vi "ScanCtrl_HR.vi"() -> ()   [LabVIEW 2020]
uses:
  C:/Users/MarcuLab/Desktop/V6 APD LV/V6 APD LV/Kinesis/Thorlabs.MotionControl.Controls.dll
  Kinesis/Thorlabs.MotionControl.Controls.dll
  <vilib>/event_ctls.llb/usereventprio.ctl
  C:/Users/MarcuLab/Desktop/V6 APD LV/V6 APD LV/Kinesis/Thorlabs.MotionControl.KCube.BrushlessMotorCLI.dll
  Kinesis/Thorlabs.MotionControl.KCube.BrushlessMotorCLI.dll
  C:/Users/MarcuLab/Desktop/V6 APD LV/V6 APD LV/Kinesis/ThorLabs.MotionControl.KCube.DCServoCLI.dll
  Kinesis/ThorLabs.MotionControl.KCube.DCServoCLI.dll
  C:/Users/MarcuLab/Desktop/V6 APD LV/V6 APD LV/Kinesis/Thorlabs.MotionControl.GenericMotorCLI.dll
  Kinesis/Thorlabs.MotionControl.GenericMotorCLI.dll
panel:
  out "error out":errorcluster
  out "TriggerPara":T1
  out "Trigger1Polarity":i32(ring)=1 items=["TriggerHigh"=1, "TriggerLow"=2]
  out "Trigger1Mode":i32(ring) items=["Disabled"=0, "TrigIN_GPI"=1, "TrigIN_RelativeMove"=2, "TrigIN_AbsoluteMove"=3, "TrigIN_Homed"=4, "TrigIN_Stop"=5, "TrigOUT_GPO"=10, "TrigOUT_InMotion"=11, "TrigOUT_AtMaxVelocity"=12, "TrigOUT_AtPositionFwd"=13, "TrigOUT_AtPositionRev"=14, "TrigOUT_AtPositionBoth"=15, "TrigOut_AtFwdLimit"=16, "TrigOut_AtBwdLimit"=17, "TrigOut_AtLimit"=18]
  in  "acceleration (mm/s2)":dbl=4000.0
  out "ScanRoute":cluster{dbl[], dbl[]}(graph)
  out "# of lines":u32
  in  "Start Scan":bool
  in  "Comp Scan Para":bool
  out "X speed (mm/s)":dbl format="%.4g"
  in  "Laser Rate (Hz)":u16=2500
  in  "Y step size (um)":dbl=10.0
  in  "X step size (um)":dbl=10.0
  in  "Y scan distance (mm)":dbl=0.2
  in  "X scan distance (mm)":dbl=30.0
  out "Y0 Position(mm)":dbl format="%.4g"
  out "GetPositionCounter 2":i32
  out "X0 Position(mm)":dbl format="%.4g"
  out "GetPositionCounter":i32
  in  "SetScanStart":bool
  in  "SerialNumber(Slow)":string="27000986"
  in  "SerialNumber(Fast)":string="28252795"
  in  "SlowAxis":refnum<k24>(container)
  in  "FastAxis":refnum<k24>(container)
  in  "Quit":bool
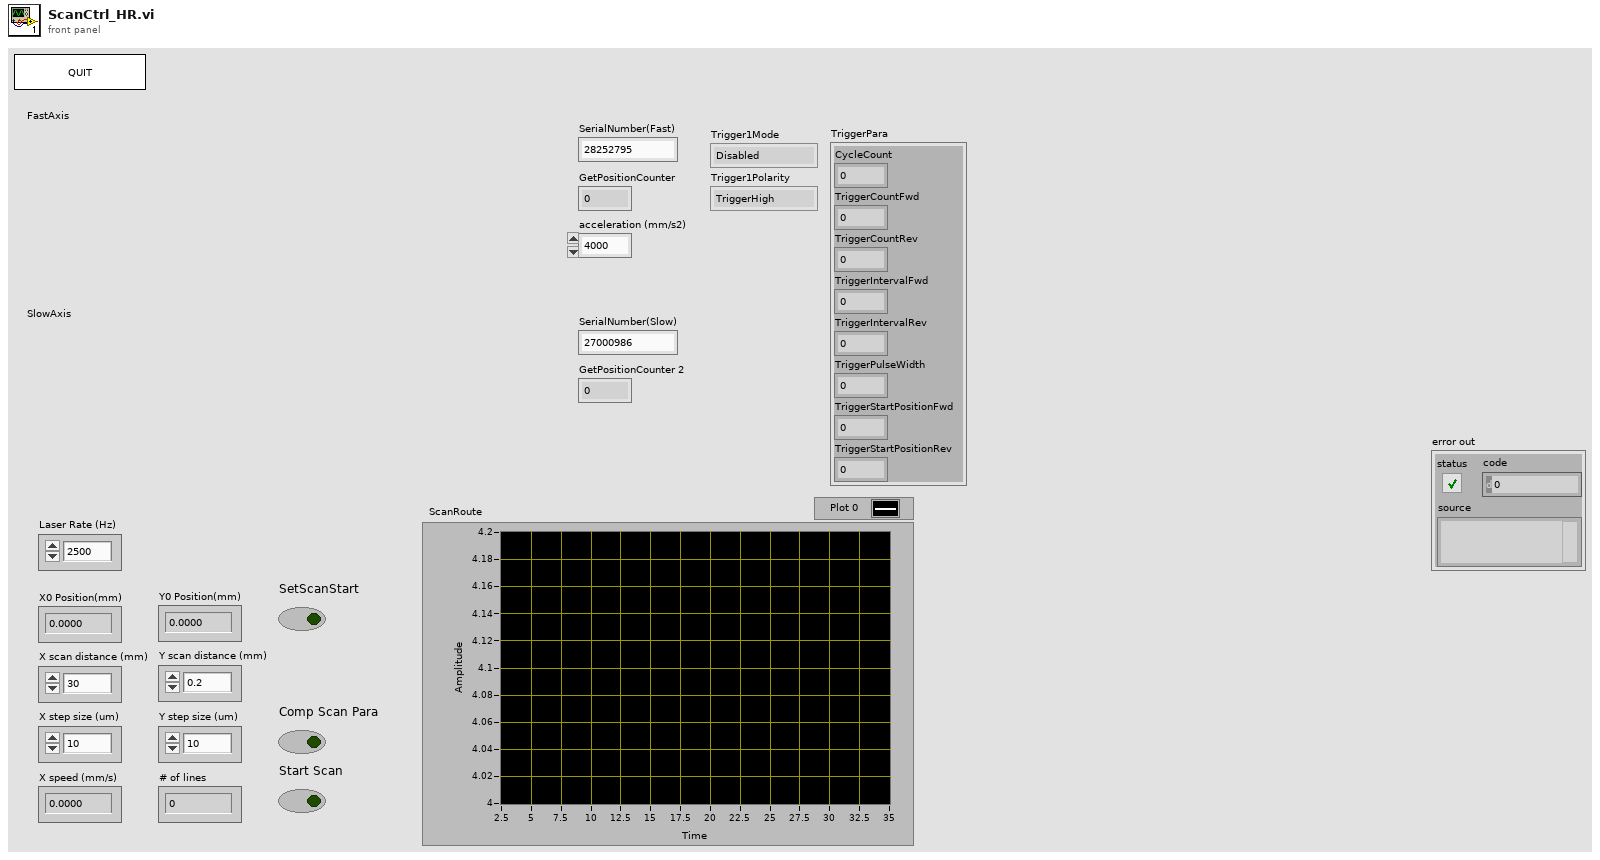
[diagram p1: front panel]
types:
  T1 = cluster{"CycleCount":i32, "TriggerCountFwd":i32, "TriggerCountRev":i32, "TriggerIntervalFwd":dbl, "TriggerIntervalRev":dbl, "TriggerPulseWidth":i32, "TriggerStartPositionFwd":dbl, "TriggerStartPositionRev":dbl}
  T2 = cluster{"X":dbl[], "Y":dbl[], "Device(Fast)":refnum<k24>, "Device(Slow)":refnum<k24>}
  T3 = enum32{"Invalid", "Standard", "Closed", "Hidden", "Minimized", "Maximized"}
  T4 = enum32{"invalid app kind", "Development System", "Run Time System", "Student Edition", "Embedded LabVIEW", "Evaluation", "Custom"}
  T5 = typedef "usereventprio.ctl" = enum32{"high priority", "normal priority"}
  T6 = enum16{"open", "open or create", "create or replace", "create", "open (read-only)"}
  T7 = cluster{"Core":cluster{"Current VI Reference":refnum<vi>, "Close Panel on Exit?":bool}, "FastAxisSerial":string, "SlowAxisSerial":string, "NetHandle(Fast)":refnum<k24>, "Device(Fast)":refnum<k24>, "NetHandle(Slow)":refnum<k24>, "Device(Slow)":refnum<k24>, "ScanRoute":cluster{dbl[], dbl[]}}
  T8 = cluster{"Current VI Reference":refnum<vi>, "Close Panel on Exit?":bool}
  T9 = cluster{"remote start event":refnum<user-event>, "remote stop event":refnum<user-event>}
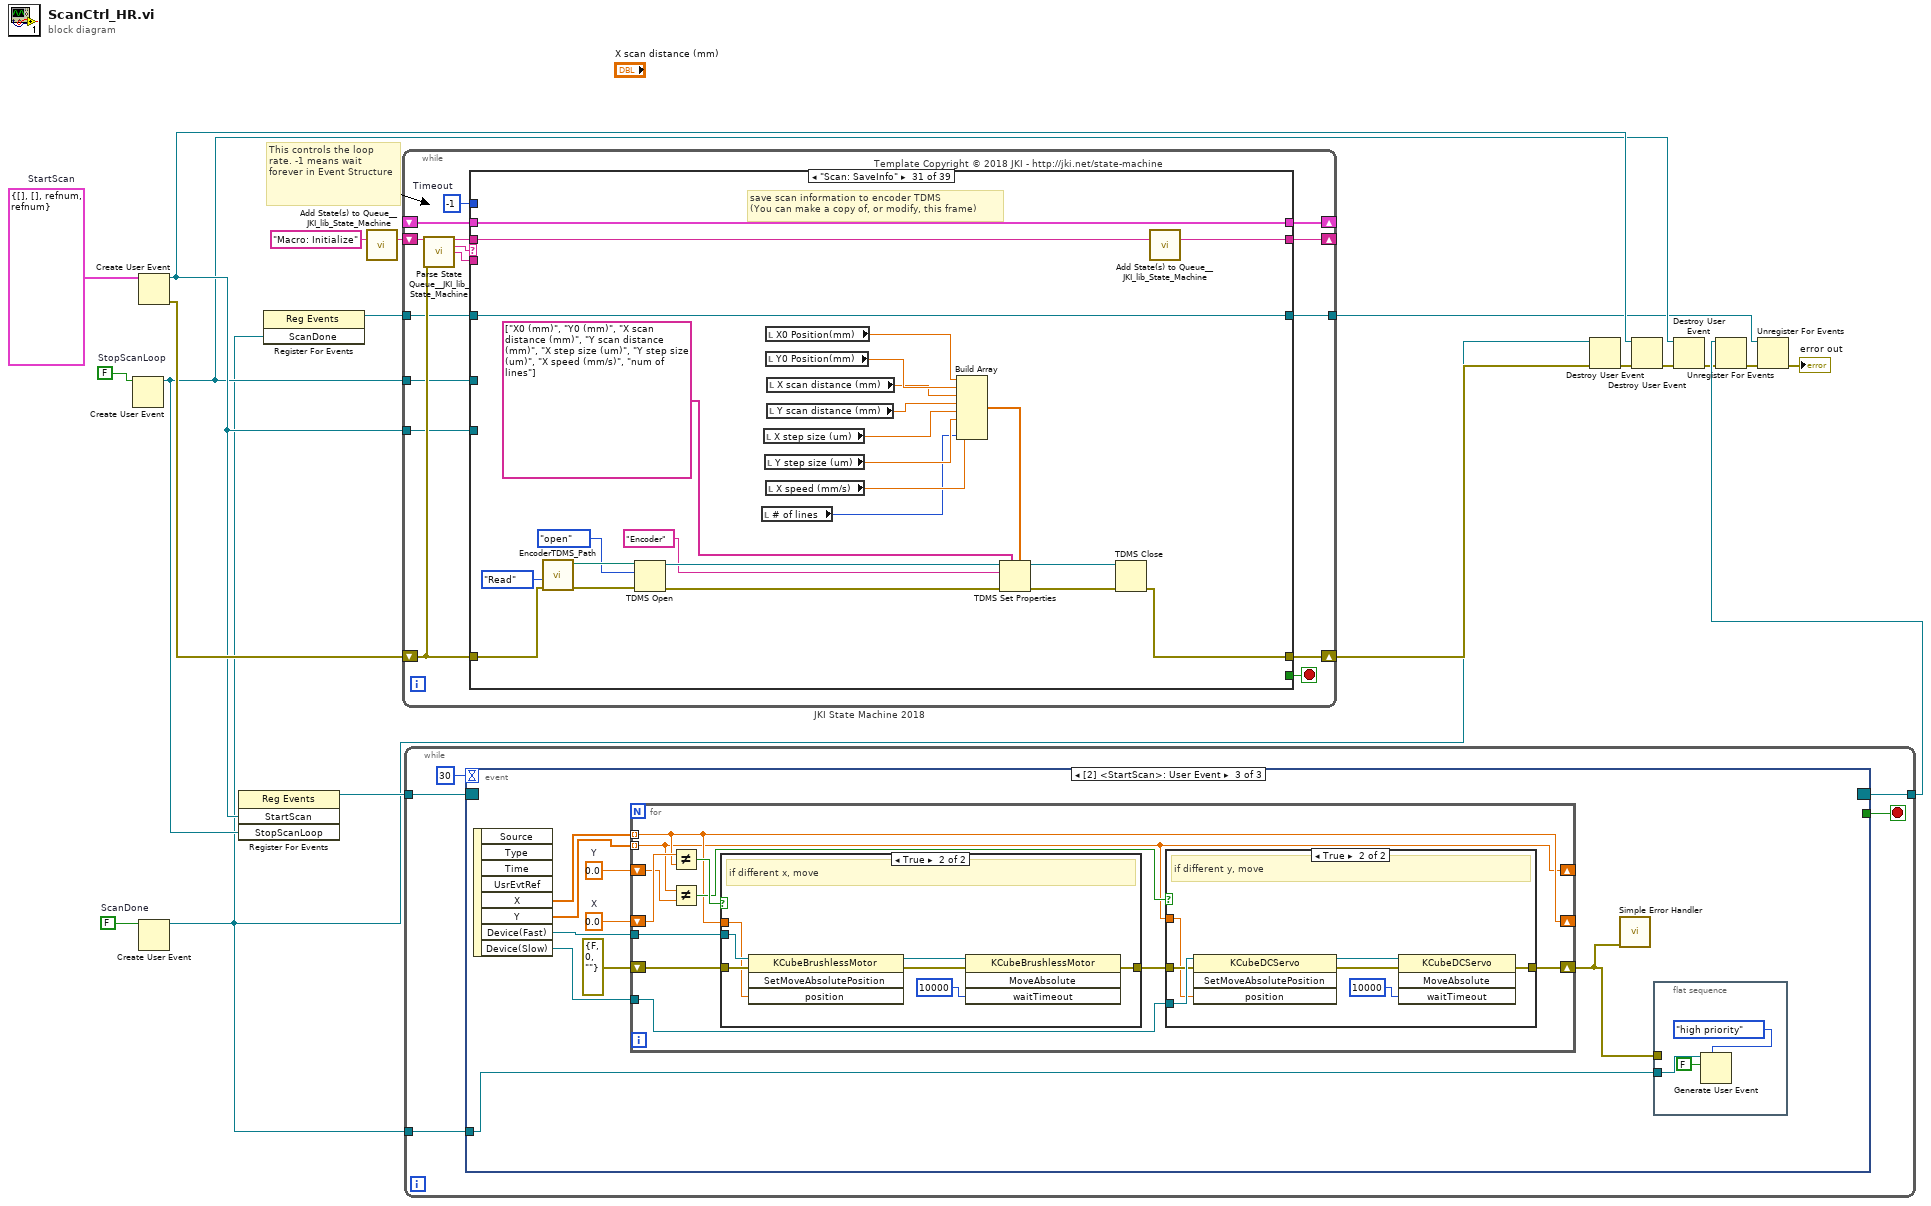
[diagram p0: block diagram]
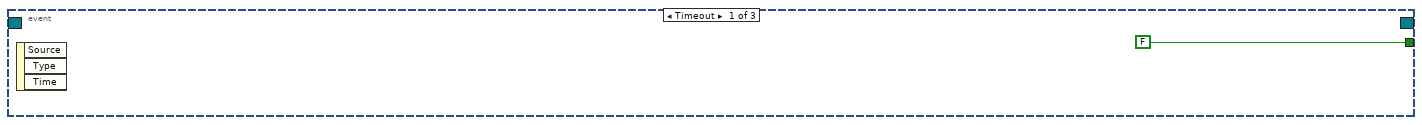
[diagram p2: hidden frame]
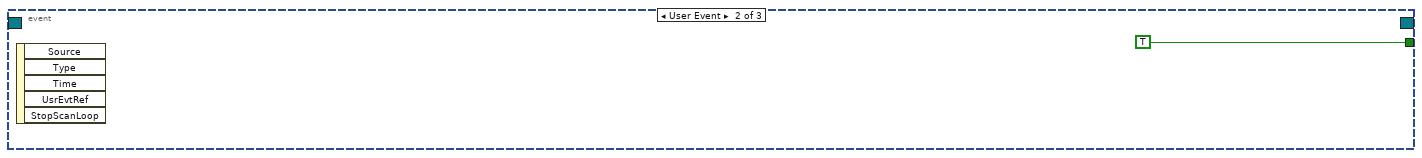
[diagram p3: hidden frame]
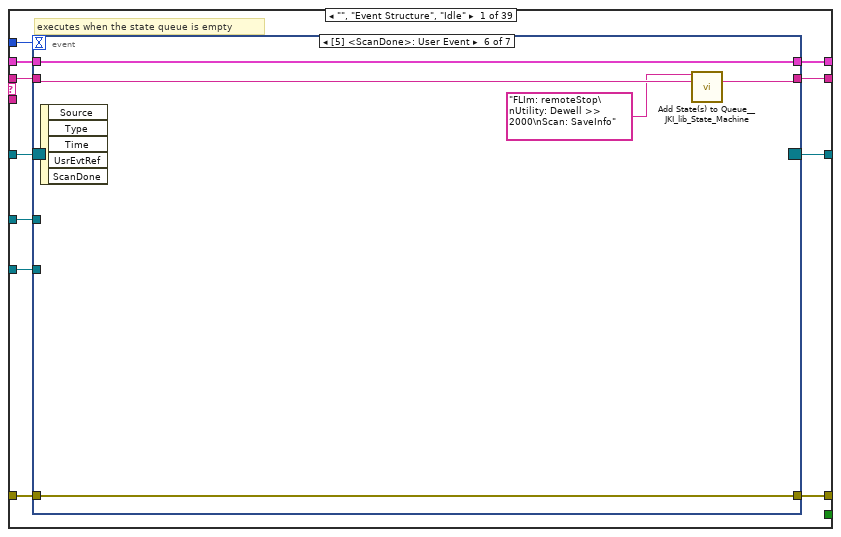
[diagram p6: hidden frame]
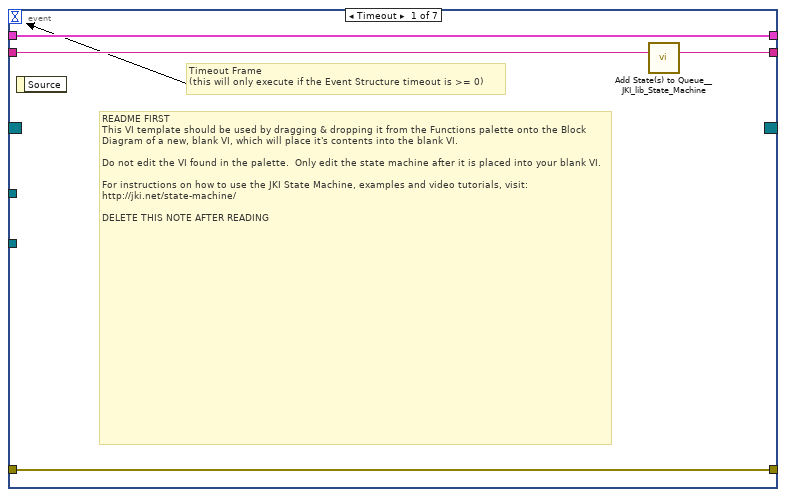
[diagram p7: hidden frame]
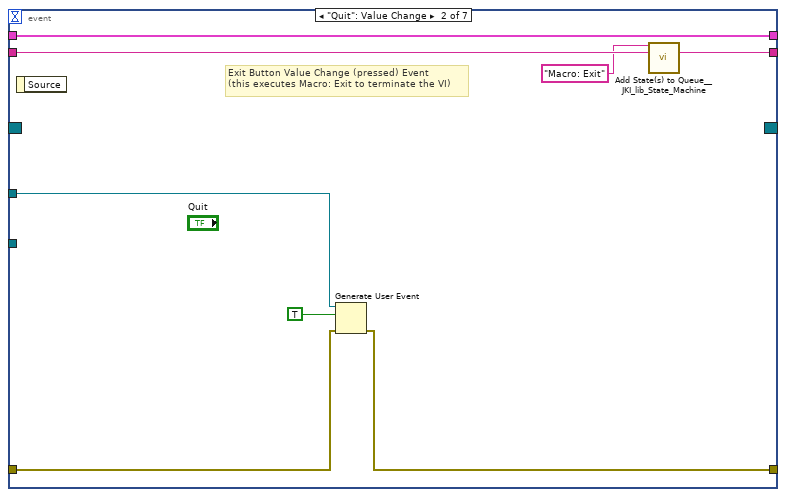
[diagram p8: hidden frame]
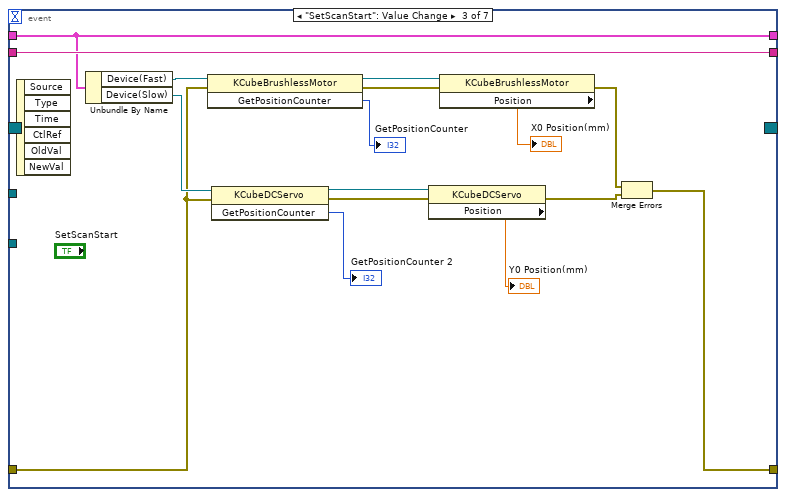
[diagram p9: hidden frame]
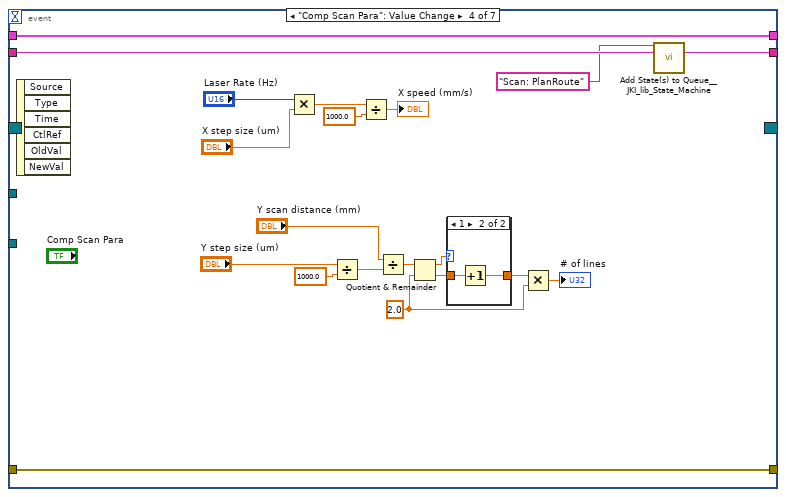
[diagram p10: hidden frame]
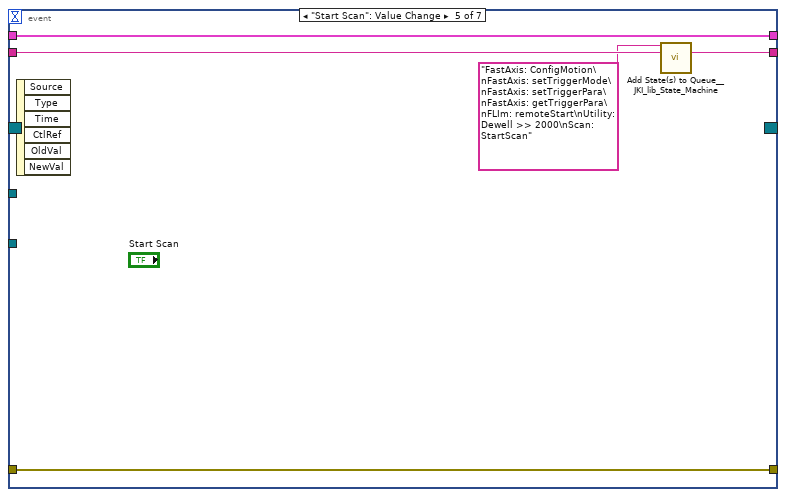
[diagram p12: hidden frame]
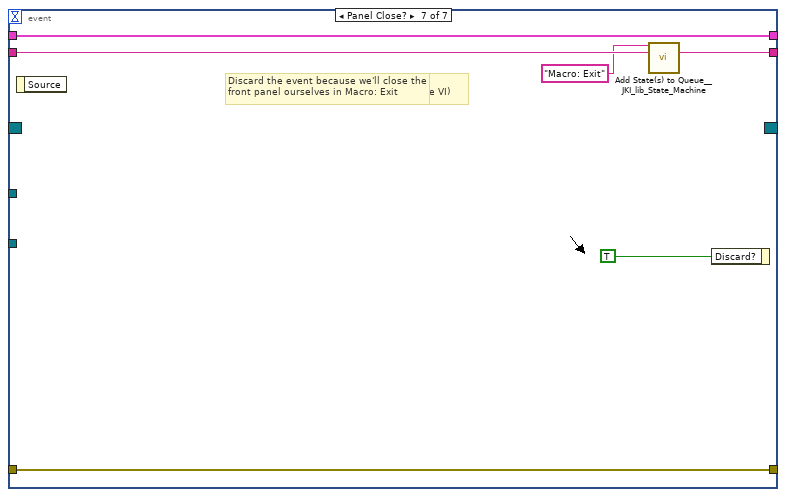
[diagram p13: hidden frame]
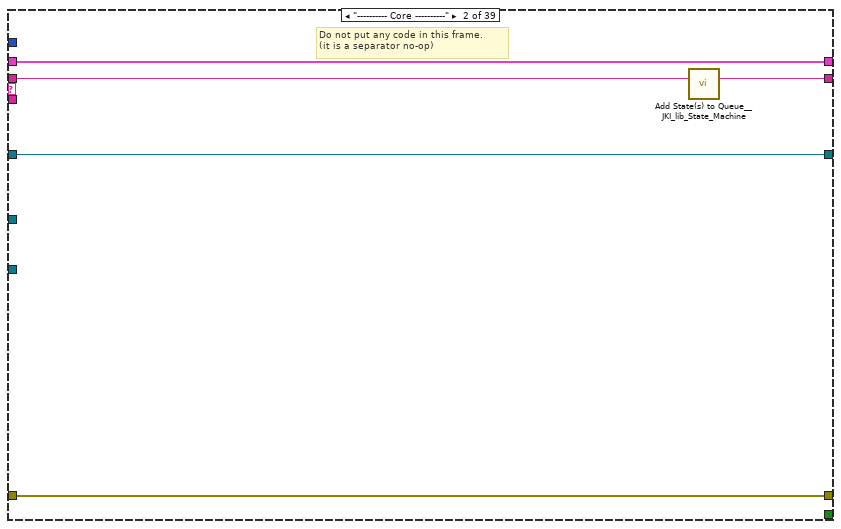
[diagram p14: hidden frame]
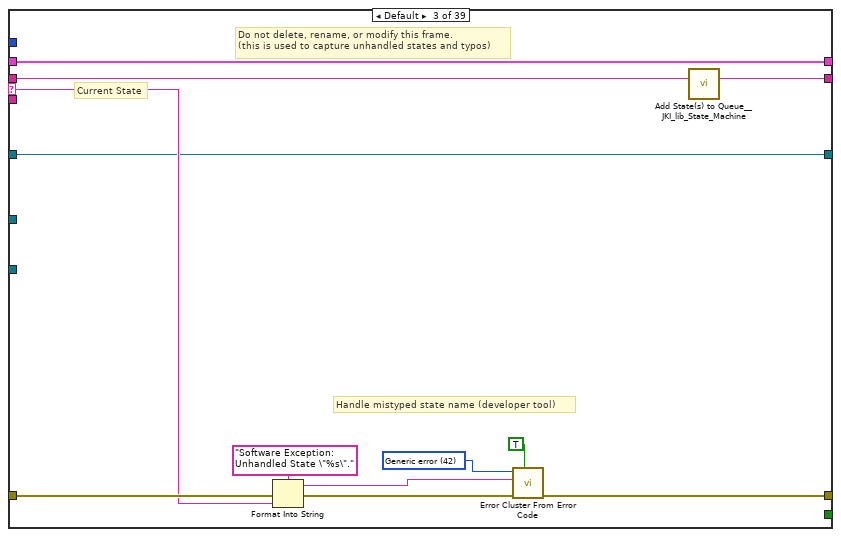
[diagram p15: hidden frame]
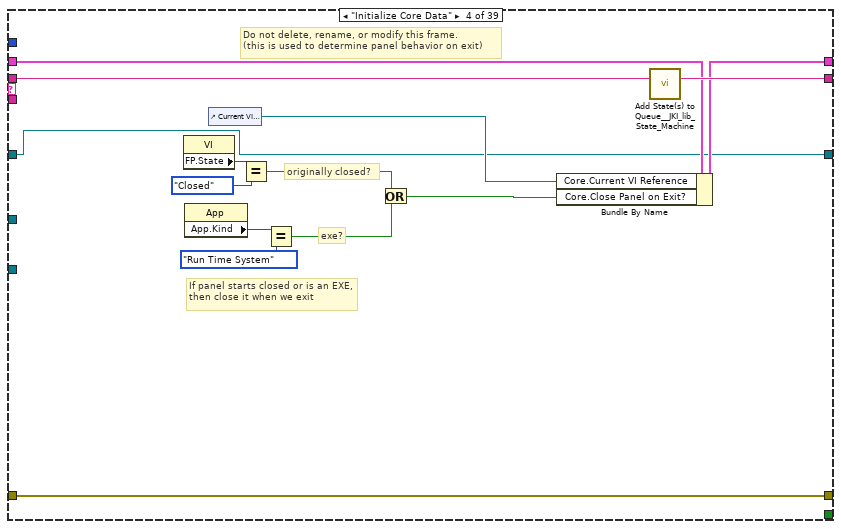
[diagram p16: hidden frame]
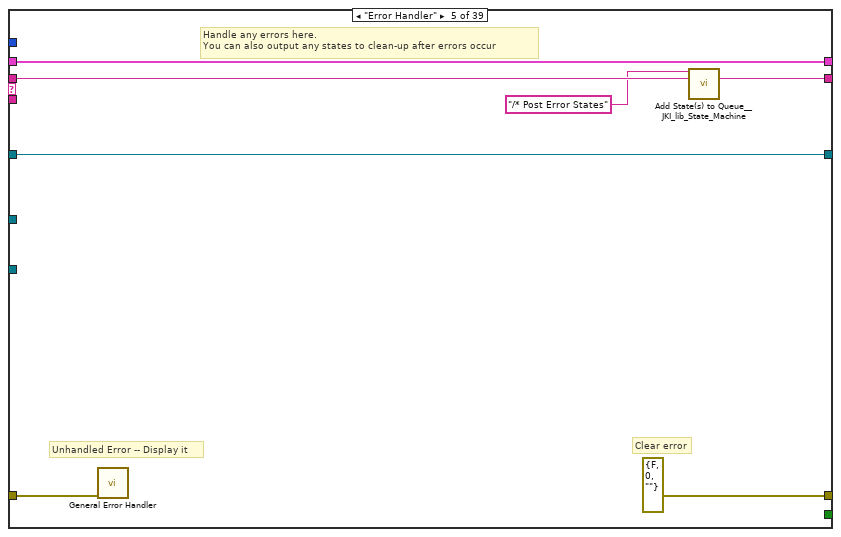
[diagram p17: hidden frame]
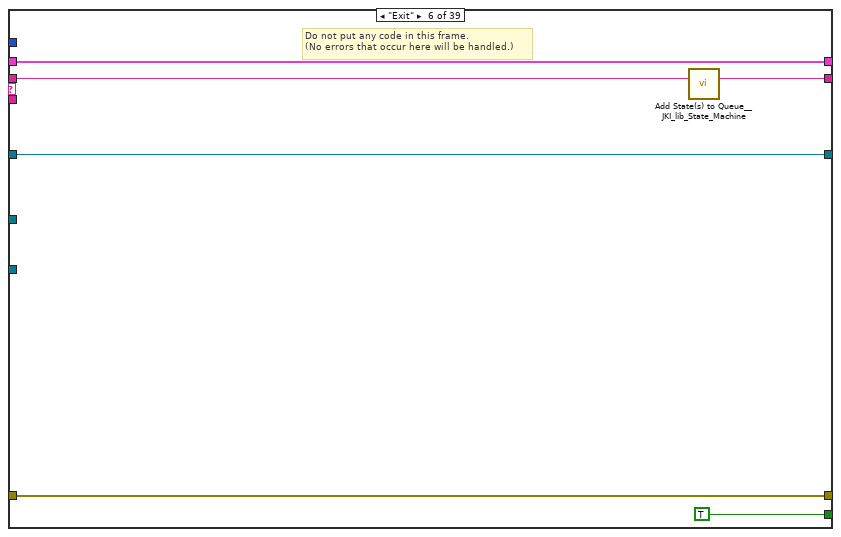
[diagram p18: hidden frame]
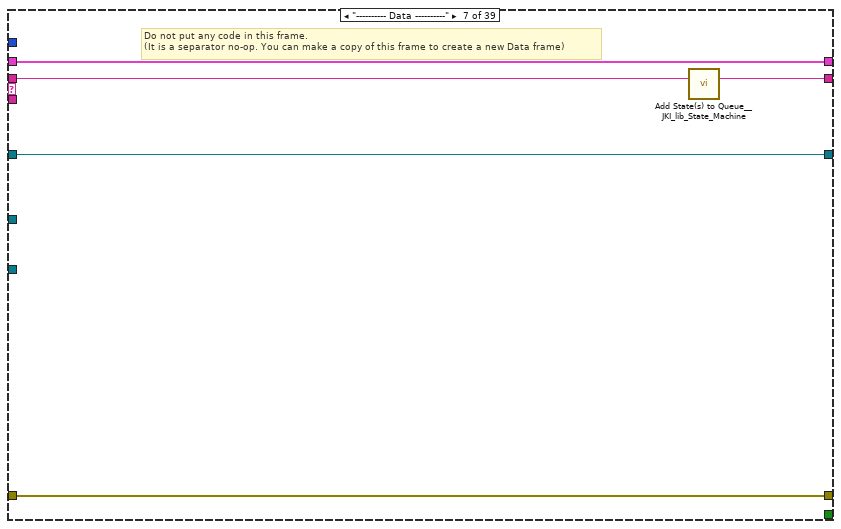
[diagram p19: hidden frame]
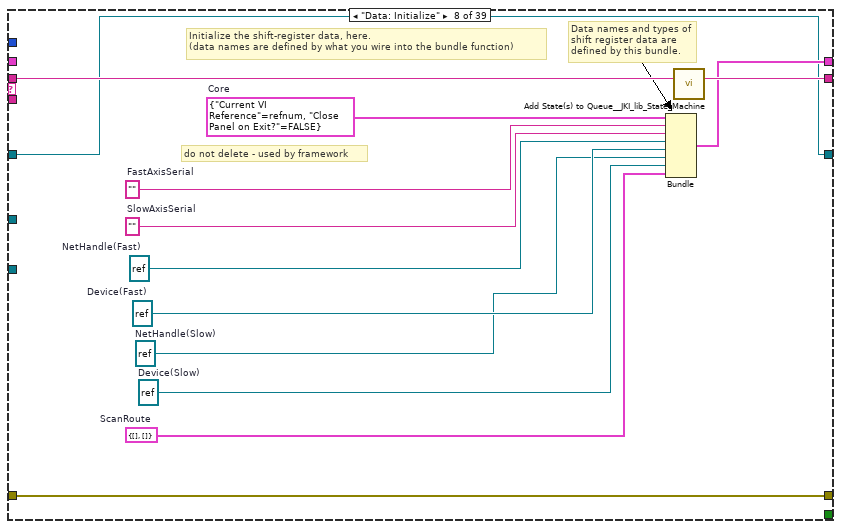
[diagram p20: hidden frame]
diagram:
  w13 = FALSE  # ScanDone
  w14 = T2 {"X"=[], "Y"=[], "Device(Fast)"=refnum, "Device(Slow)"=refnum}  # StartScan
  w15 = FALSE  # StopScanLoop
  # "This controls the loop rate. -1 means wait forever in Event Structure"
  n1 = Create User Event(user event datatype=w15) -> (user event=w10:refnum<user-event>)  [unwired: 1 in, 1 out]
  n2 = Create User Event(user event datatype=w14) -> (user event=w11:refnum<user-event>, error out=w16:errorcluster)  [unwired: 1 in]
  n3 = Create User Event(user event datatype=w13) -> (user event=w4:refnum<user-event>)  [unwired: 1 in, 1 out]
  n4 = register-events(w11, w10) -> (reference out=w17:refnum<event-registration>)  [unwired: 2 in, 1 out]
  n5 = register-events(w4) -> (reference out=w5:refnum<event-registration>)  [unwired: 2 in, 1 out]
  n6 = call <vilib>:"Add State(s) to Queue__JKI_lib_State_Machine.vi"("State(s) in (\"\")"="Macro: Initialize") -> ("States Out"=w19:string)  [unwired: 14 in]
  n7 = while "JKI State Machine 2018" {
    shift-right: [w27] -> _
    shift-left: _ -> [w26]
    shift-right: [w30] -> w6
    shift-left: w16 -> [w24]
    shift-right: [w29] -> _
    shift-left: w19 -> [w31]
    tunnel: w10 -> [w23]
    tunnel: w11 -> [w22]
    tunnel: w5 -> [w21]
    tunnel: [w20] -> w1
    stop <- w28 stop-if-true
    w25 = -1  # Timeout
    # "Template Copyright © 2018 JKI - http://jki.net/state-machine"
    n8 = call <vilib>:"Parse State Queue__JKI_lib_State_Machine.vi"("State Queue"=w31, "Error In (no error)"=w24) -> ("Remaining States"=w33:string, "Current State"=w34:string, "Arguments"=w32:string)  [unwired: 11 in]
    n9 = case shown="\"Scan: SaveInfo\"" w34 {
      selector: w34 -> [_ _ w119 _ _ _ _ _ _ _ _ _ _ _ _ _ _ _ _ _ _ _ _ _ _ _ _ _ _ _ _ _ _ _ _ _ _ _ _]
      tunnel: w33 -> [w45 w117 w123 w143 w150 w156 w161 w174 w181 w186 w191 w198 w210 w280 w286 w298 w303 w321 w330 w337 w373 w397 w404 w409 w422 w427 w434 w439 w451 w492 w517 w522 w533 w544 w549 w556 w561 w566 w571]
      tunnel: w32 -> [_ _ _ _ _ _ _ _ _ _ _ w193 w204 _ _ _ _ _ _ _ _ _ _ _ _ _ _ _ _ _ _ _ _ _ _ w552 _ _ _]
      tunnel: w26 -> [w43 w114 w121 w136 w147 w154 w158 _ w176 w183 w189 w196 w206 w277 w283 w295 w300 w313 w328 w335 w371 w395 w402 w406 w419 w424 w432 w436 w442 w482 w515 w519 w532 w542 w546 w553 w558 w563 w568]
      tunnel: [w42 w115 w125 w140 errorcluster {"status"=FALSE, "code"=0, "source"=""} ("error out") w153 w159 w171 w177 w184 w188 w194 w207 w278 w284 w296 w301 w306 w324 w333 w362 w376 w400 w407 w412 w425 w429 w437 w450 w480 w494 w520 w525 w536 w547 w554 w559 w564 w569] -> w30
      tunnel: w24 -> [w41 w115 w124 w140 w146 w153 w159 w171 w178 w184 w188 w195 w208 w278 w284 w296 w301 w317 w323 w332 w361 w375 w400 w407 w411 w425 w429 w437 w450 w479 w493 w520 w524 w535 w547 w554 w559 w564 w569]
      tunnel: [w44 w116 w122 w142 w149 w155 w160 w173 w180 w185 w190 w197 w209 w279 w285 w297 w302 w321 w329 w336 w372 w396 w403 w408 w422 w426 w433 w438 w451 w491 w516 w521 w533 w543 w548 w555 w560 w565 w570] -> w29
      tunnel: [_ _ _ _ _ TRUE _ _ _ _ _ _ _ _ _ _ _ _ _ _ _ _ _ _ _ _ _ _ _ _ _ _ _ _ _ _ _ _ _] -> w28
      tunnel: [w40 w114 w121 w141 w147 w154 w158 w172 w176 w183 w189 w196 w206 w277 w283 w295 w300 w314 w328 w335 w371 w395 w402 w406 w418 w424 w432 w436 w443 w482 w515 w519 w532 w542 w546 w553 w558 w563 w568] -> w27
      tunnel: w25 -> [w39 _ _ _ _ _ _ _ _ _ _ _ _ _ _ _ _ _ _ _ _ _ _ _ _ _ _ _ _ _ _ _ _ _ _ _ _ _ _]
      tunnel: w23 -> [w38 _ _ _ _ _ _ _ _ _ _ _ _ _ _ _ _ _ _ _ _ _ _ _ _ _ _ _ _ _ _ _ _ _ _ _ _ _ _]
      tunnel: w22 -> [w37 _ _ _ _ _ _ _ _ _ _ _ _ _ _ _ _ _ _ _ _ _ _ _ _ _ _ _ _ w481 _ _ _ _ _ _ _ _ _]
      tunnel: w21 -> [w36 w113 w118 w130 w144 w151 w157 w162 w175 w182 w187 w192 w203 w276 w281 w287 w299 w304 w322 w331 w358 w374 w398 w405 w410 w423 w428 w435 w440 w478 w514 w518 w523 w534 w545 w550 w557 w562 w567]
      tunnel: [w35 w113 w118 w130 w144 w151 w157 w162 w175 w182 w187 w192 w203 w276 w281 w287 w299 w304 w322 w331 w358 w374 w398 w405 w410 w423 w428 w435 w440 w478 w514 w518 w523 w534 w545 w550 w557 w562 w567] -> w20
      frame "", "Event Structure", "Idle" {
        # "executes when the state queue is empty"
        n10 = event shown="[5] <ScanDone>: User Event" {
          selector: w36 -> [_ _ _ _ _ _ _]
          dyn-events: [_ _ _ _ _ _ _] -> w35
          timeout: w39 -> [_ _ _ _ _ _ _]
          tunnel: w45 -> [w49 w57 w73 w75 w99 w104 w112]
          tunnel: [w48 w56 w73 w76 w100 w103 w111] -> w44
          tunnel: w43 -> [w46 w55 w67 w87 w101 w105 w109]
          tunnel: [w47 w51 w58 w88 w97 w106 w110] -> w42
          tunnel: w41 -> [w47 w50 w65 w88 w97 w106 w110]
          tunnel: [w46 w55 w67 w87 w101 w105 w109] -> w40
          tunnel: w38 -> [_ w53 _ _ _ _ _]
          tunnel: w37 -> [_ _ _ _ _ _ _]
          event Timeout {
            # "README FIRST\nThis VI template should be used by dragging & dropping it from the Functions palette onto the Block Diagram of a new, blank VI, which will place it's contents into the blank VI.\n\nDo not edit the VI found in the palette.  Only edit the state machine after it is placed into your blank VI.\n\nFor instructions on how to use the JKI State Machine, examples and video tutorials, visit:\nhttp://jki.net/state-machine/\n\nDELETE THIS NOTE AFTER READING"
            # "Timeout Frame\n(this will only execute if the Event Structure timeout is >= 0)"
            n11 = event-data() -> ()  [unwired: 1 in, 1 out]
            n12 = call <vilib>:"Add State(s) to Queue__JKI_lib_State_Machine.vi"("State(s) in (\"\")"=w49) -> ("States Out"=w48:string)  [unwired: 14 in]
          }
          event "Quit": Value Change {
            # "Exit Button Value Change (pressed) Event\n(this executes Macro: Exit to terminate the VI)"
            n13 = event-data() -> ()  [unwired: 1 in, 1 out]
            n14 = Generate User Event(user event=w53, event data cluster=TRUE ("event data"), error in=w50) -> (error out=w51:errorcluster)  [unwired: 1 in, 1 out]
            n15 = call <vilib>:"Add State(s) to Queue__JKI_lib_State_Machine.vi"("State(s) in Front (\"\")"="Macro: Exit", "State(s) in (\"\")"=w57) -> ("States Out"=w56:string)  [unwired: 13 in]
          }
          event "SetScanStart": Value Change {
            n16 = event-data() -> ()  [unwired: 1 in, 6 out]
            n17 = Unbundle By Name(w67) -> ("Device(Fast)"=w72:refnum<k24>, "Device(Slow)"=w66:refnum<k24>)
            n18 = invoke class="KCubeBrushlessMotor" method="GetPositionCounter"(reference=w72, error in=w65) -> (reference out=w69:refnum<k24>, error out=w68:errorcluster, "GetPositionCounter"=→"GetPositionCounter":i32)  [unwired: 1 in]
            n19 = invoke class="KCubeDCServo" method="GetPositionCounter"(reference=w66, error in=w65) -> (reference out=w63:refnum<k24>, error out=w62:errorcluster, "GetPositionCounter"=→"GetPositionCounter 2":i32)  [unwired: 1 in]
            n20 = property class="KCubeDCServo"(reference=w63, error in=w62) -> (error out=w60:errorcluster, "Position"=→"Y0 Position(mm)":dbl)  [unwired: 1 out]
            n21 = property class="KCubeBrushlessMotor"(reference=w69, error in=w68) -> (error out=w59:errorcluster, "Position"=→"X0 Position(mm)":dbl)  [unwired: 1 out]
            n22 = Merge Errors(w59, w60) -> (w58:errorcluster)
          }
          event "Comp Scan Para": Value Change {
            w81 = 2.0 ("y")
            n23 = event-data() -> ()  [unwired: 1 in, 6 out]
            n24 = Multiply(x="Laser Rate (Hz)", y="X step size (um)") -> (x*y=w91:dbl)
            n25 = Divide(x="Y step size (um)", y=1000.0) -> (x/y=w84:dbl)
            n26 = Divide(x=w91, y=1000.0) -> (x/y=→"X speed (mm/s)":dbl)
            n27 = Divide(x="Y scan distance (mm)", y=w84) -> (x/y=w83:dbl)
            n28 = Quotient & Remainder(x=w83, y=w81) -> (x-y*floor(x/y)=w79:dbl, floor(x/y)=w78:dbl)
            n29 = case shown="1" w79 {
              tunnel: w78 -> [w94 w96]
              tunnel: [w94 w95] -> w77
              frame 0, Default {
              }
              frame 1 {
                n30 = Increment(x=w96) -> (x+1=w95:dbl)
              }
            }
            n31 = Multiply(x=w77, y=w81) -> (x*y=→"# of lines":dbl)
            n32 = call <vilib>:"Add State(s) to Queue__JKI_lib_State_Machine.vi"("State(s) in Front (\"\")"="Scan: PlanRoute" ("State(s) in Front (\"\")"), "State(s) in (\"\")"=w75) -> ("States Out"=w76:string)  [unwired: 13 in]
          }
          event "Start Scan": Value Change {
            n33 = event-data() -> ()  [unwired: 1 in, 6 out]
            n34 = call <vilib>:"Add State(s) to Queue__JKI_lib_State_Machine.vi"("State(s) in Front (\"\")"="FastAxis: ConfigMotion\nFastAxis: setTriggerMode\nFastAxis: setTriggerPara\nFastAxis: getTriggerPara\nFLIm: remoteStart\nUtility: Dewell >> 2000\nScan: StartScan" ("State(s) in Front (\"\")"), "State(s) in (\"\")"=w99) -> ("States Out"=w100:string)  [unwired: 13 in]
          }
          event User Event {
            n35 = event-data() -> ()  [unwired: 1 in, 5 out]
            n36 = call <vilib>:"Add State(s) to Queue__JKI_lib_State_Machine.vi"("State(s) in Front (\"\")"="FLIm: remoteStop\nUtility: Dewell >> 2000\nScan: SaveInfo" ("State(s) in Front (\"\")"), "State(s) in (\"\")"=w104) -> ("States Out"=w103:string)  [unwired: 13 in]
          }
          event Panel Close? {
            # "Discard the event because we'll close the front panel ourselves in Macro: Exit"
            # "Close Panel button (pressed) Event\n(this executes Macro: Exit to terminate the VI)"
            n37 = event-data() -> ()  [unwired: 1 in, 1 out]
            n38 = call <vilib>:"Add State(s) to Queue__JKI_lib_State_Machine.vi"("State(s) in Front (\"\")"="Macro: Exit", "State(s) in (\"\")"=w112) -> ("States Out"=w111:string)  [unwired: 13 in]
            n39 = event-data("Discard?"=TRUE) -> ()  [unwired: 1 in, 1 out]
          }
        }
      }
      frame "---------- Core ----------" {
        # "Do not put any code in this frame.\n(it is a separator no-op)"
        n40 = call <vilib>:"Add State(s) to Queue__JKI_lib_State_Machine.vi"("State(s) in (\"\")"=w117) -> ("States Out"=w116:string)  [unwired: 14 in]
      }
      frame Default {
        w128 = 42 items=["No error", "Argument error", "Memory is full", "Out of zone", "End of file", "File already open", "Generic file I/O error", "File not found", "File permission error", "Disk is full", "Duplicate path", "Too many files open", "System feature not enabled", "Resource file not found", "Cannot add resource", "Resource not found", "Image not found", "Image memory error", "Pen does not exist", "Config type invalid", "Config token not found", "Config parse error", "Config memory error", "Bad external code format", "Bad external code offset", "External code not present", "Null window", "Destroy window error", "Null menu", "Print aborted", "Bad print record", "Print driver error", "Windows error during printing", "Memory error during printing", "Print dialog error", "Generic print error", "Invalid device refnum", "Device not found", "Device parameter error", "Device unit error", "Cannot open device", "Device call aborted", "Generic error", "Cancelled by user", "Object ID too low", "Object ID too high", "Object not in heap", "Unknown heap", "Unknown object (invalid DefProc)", "Unknown object (DefProc not in table)", "Message out of range", "Invalid (null) method", "Unknown message", "Manager call not supported", "Bad address", "Network operation in progress", "Network operation timed out", "Connection is busy", "Network attribute not supported", "Network error", "Address in use", "System out of memory", "Connection aborted", "Connection refused", "Not connected", "Already connected", "Connection closed", "Initialization error (interapplication manager)", "Bad occurrence", "Wait on unbound occurrence handler", "Occurrence queue overflow", "Datalog type conflict", "Unused", "Unrecognized type (interapplication manager)", "Memory corrupt", "Failed to make temporary DLL", "Old CIN version", "Drag socket not found", "Failed to load drop-object", "Failed to register OLE object", "Failed to release OLE object", "Format specifier type mismatch", "Unknown format specifier", "Too few format specifiers", "Too many format specifiers", "Scan failed", "Newer CIN version", "Error converting to variant", "Runtime menu error", "Password tampered", "Variant attribute not found", "Incompatible variant data type", "Event data is not available", "Event Store is not present", "Occurrence is not found", "Event Queue is not created", "Event info is not available", "Refnum passed is NULL", "Error retrieving Class GUID", "Error retrieving CoClass GUID", "Error retrieving TypeLib GUID.", "Bad built application magic bytes.", "Specific driver is different from the specific driver associated with the Logical Name.", "There is no session opened to the class driver.", "Max Error", "MAX - Error with config objects", "MAX - Error loading configuration", "MAX - Group not supported"]
        # "Current State"
        # "Do not delete, rename, or modify this frame.\n(this is used to capture unhandled states and typos)"
        # "Handle mistyped state name (developer tool)"
        n41 = Format Into String(format string="Software Exception: Unhandled State \"%s\"." ("message"), error in=w124, w119) -> (resulting string=w127:string, error out=w126:errorcluster)  [unwired: 1 in]
        n42 = call <vilib>:"Error Cluster From Error Code.vi"("show call chain? (False)"=TRUE, "error in (no error)"=w126, "error message (\"\")"=w127, "error code (0)"=w128) -> ("error out"=w125:errorcluster)  [unwired: 5 in]
        n43 = call <vilib>:"Add State(s) to Queue__JKI_lib_State_Machine.vi"("State(s) in (\"\")"=w123) -> ("States Out"=w122:string)  [unwired: 14 in]
      }
      frame "Initialize Core Data" {
        # "Do not delete, rename, or modify this frame.\n(this is used to determine panel behavior on exit)"
        # "originally closed?"
        # "exe?"
        # "If panel starts closed or is an EXE, then close it when we exit"
        n44 = property class="VI"() -> ("FP.State"=w133:T3)  [unwired: 2 in, 2 out]
        n45 = property class="App"() -> ("App.Kind"=w139:T4)  [unwired: 2 in, 2 out]
        n46 = control-ref of="Current VI Reference"() -> (w134:refnum<vi>)
        n47 = Equal?(x=w133, y=T3."Closed" ("Front Panel Window:State")) -> (x = y?=w131:bool)
        n48 = Equal?(x=w139, y=T4."Run Time System" ("Application:Kind")) -> (x = y?=w137:bool)
        n49 = Or(x=w131, y=w137) -> (x .or. y?=w135:bool)
        n50 = Bundle By Name(cluster=w136, "Core.Current VI Reference"=w134, "Core.Close Panel on Exit?"=w135) -> (w141:T7)
        n51 = call <vilib>:"Add State(s) to Queue__JKI_lib_State_Machine.vi"("State(s) in (\"\")"=w143) -> ("States Out"=w142:string)  [unwired: 14 in]
      }
      frame "Error Handler" {
        # "Unhandled Error -- Display it"
        # "Handle any errors here.\nYou can also output any states to clean-up after errors occur"
        # "Clear error"
        n52 = call <vilib>:"General Error Handler.vi"("error in (no error)"=w146) -> ()  [unwired: 10 in, 5 out]
        n53 = call <vilib>:"Add State(s) to Queue__JKI_lib_State_Machine.vi"("State(s) in Front (\"\")"="/* Post Error States", "State(s) in (\"\")"=w150) -> ("States Out"=w149:string)  [unwired: 13 in]
      }
      frame "Exit" {
        # "Do not put any code in this frame.\n(No errors that occur here will be handled.)"
        n54 = call <vilib>:"Add State(s) to Queue__JKI_lib_State_Machine.vi"("State(s) in (\"\")"=w156) -> ("States Out"=w155:string)  [unwired: 14 in]
      }
      frame "---------- Data ----------" {
        # "Do not put any code in this frame.\n(It is a separator no-op. You can make a copy of this frame to create a new Data frame)"
        n55 = call <vilib>:"Add State(s) to Queue__JKI_lib_State_Machine.vi"("State(s) in (\"\")"=w161) -> ("States Out"=w160:string)  [unwired: 14 in]
      }
      frame "Data: Initialize" {
        w163 = cluster{dbl[], dbl[]} {[], []}  # ScanRoute
        w164 = refnum<k24> refnum  # Device(Slow)
        w165 = refnum<k24> refnum  # NetHandle(Slow)
        w166 = refnum<k24> refnum  # NetHandle(Fast)
        w167 = refnum<k24> refnum  # Device(Fast)
        w168 = ""  # SlowAxisSerial
        w169 = T8 {"Current VI Reference"=refnum, "Close Panel on Exit?"=FALSE}  # Core
        w170 = ""  # FastAxisSerial
        # "do not delete - used by framework"
        # "Data names and types of shift register data are defined by this bundle."
        # "Initialize the shift-register data, here.\n(data names are defined by what you wire into the bundle function)"
        n56 = Bundle("Core"=w169, "FastAxisSerial"=w170, "SlowAxisSerial"=w168, "NetHandle(Fast)"=w166, "Device(Fast)"=w167, "NetHandle(Slow)"=w165, "Device(Slow)"=w164, "ScanRoute"=w163) -> (w172:T7)  [unwired: 1 in]
        n57 = call <vilib>:"Add State(s) to Queue__JKI_lib_State_Machine.vi"("State(s) in (\"\")"=w174) -> ("States Out"=w173:string)  [unwired: 14 in]
      }
      frame "Data: Cleanup" {
        # "Cleanup any data and references, here.\n(this is called automatically, by the Macro: Exit)"
        n58 = Unbundle By Name(w176) -> ("Core.Current VI Reference"=w179:refnum<vi>)
        n59 = Close Reference(reference=w179, error in (no error)=w178) -> (error out=w177:errorcluster)
        n60 = call <vilib>:"Add State(s) to Queue__JKI_lib_State_Machine.vi"("State(s) in (\"\")"=w181) -> ("States Out"=w180:string)  [unwired: 14 in]
      }
      frame "---------- UI ----------" {
        # "Do not put any code in this frame.\n(It is a separator no-op. You can make a copy of this frame to create a new UI frame)"
        n61 = call <vilib>:"Add State(s) to Queue__JKI_lib_State_Machine.vi"("State(s) in (\"\")"=w186) -> ("States Out"=w185:string)  [unwired: 14 in]
      }
      frame "UI: Initialize" {
        # "Initialize the User Interface, here.\n(this is called automatically, by the Macro: Init)"
        n62 = call <vilib>:"Add State(s) to Queue__JKI_lib_State_Machine.vi"("State(s) in (\"\")"=w191) -> ("States Out"=w190:string)  [unwired: 14 in]
      }
      frame "UI: Cursor Set" {
        # "Argument"
        # "Set and Unset Cursor Busy.\n(Usage: \"UI: Cursor Set >> Busy|Idle\")"
        n63 = case shown="\"Idle\", Default" w193 {
          tunnel: w195 -> [w200 w202]
          tunnel: [w199 w201] -> w194
          frame "Idle", Default {
            n64 = call <vilib>:"Unset Busy.vi"("error in (no error)"=w200) -> ("error out"=w199:errorcluster)  [unwired: 10 in]
          }
          frame "Busy" {
            n65 = call <vilib>:"Set Busy.vi"("error in (no error)"=w202) -> ("error out"=w201:errorcluster)  [unwired: 9 in, 1 out]
          }
        }
        n66 = call <vilib>:"Add State(s) to Queue__JKI_lib_State_Machine.vi"("State(s) in (\"\")"=w198) -> ("States Out"=w197:string)  [unwired: 14 in]
      }
      frame "UI: Front Panel State" {
        # "Argument"
        # "Set Front Panel Open or Closed\n(Usage: \"UI: Front Panel State >> Open|Close\")"
        n67 = Unbundle By Name(w206) -> ("Core.Current VI Reference"=w205:refnum<vi>)
        n68 = case shown="\"Minimize\", \"Minimized\"" w204 {
          tunnel: w208 -> [w216 w231 w242 w255 w268]
          tunnel: [w218 w232 w244 w257 w270] -> w207
          tunnel: w205 -> [w217 w229 w243 w256 w269]
          frame "Open", "Standard", Default {
            w211 = T3."Standard" ("State")
            n69 = property class="VI"(reference=w217, error in=w216) -> (reference out=w214:refnum<vi>, error out=w215:errorcluster, "FP.State"=w213:T3)
            n70 = Not Equal?(x=w213, y=w211) -> (x != y?=w212:bool)
            n71 = case shown="True" w212 {
              tunnel: [w222 w224] -> w218
              tunnel: w215 -> [w221 w224]
              tunnel: w214 -> [w220 _]
              tunnel: w211 -> [w219 _]
              frame True {
                n72 = invoke class="VI" method="FP.Open"(reference=w220, error in=w221, "Activate"=TRUE, "State"=w219) -> (error out=w222:errorcluster)  [unwired: 1 in, 4 out]
              }
              frame False {
              }
            }
          }
          frame "Close", "Closed" {
            n73 = property class="VI"(reference=w229, error in=w231) -> (reference out=w228:refnum<vi>, error out=w230:errorcluster, "FP.State"=w226:T3)
            n74 = Not Equal?(x=w226, y=T3."Closed" ("Front Panel Window:State")) -> (x != y?=w225:bool)
            n75 = case shown="True" w225 {
              tunnel: [w233 w236] -> w232
              tunnel: w230 -> [w233 w235]
              tunnel: w228 -> [_ w234]
              frame False {
              }
              frame True {
                n76 = invoke class="VI" method="FP.Close"(reference=w234, error in=w235) -> (error out=w236:errorcluster)  [unwired: 1 in, 2 out]
              }
            }
          }
          frame "Hidden", "Hide" {
            w237 = T3."Hidden" ("State")
            n77 = property class="VI"(reference=w243, error in=w242) -> (reference out=w240:refnum<vi>, error out=w241:errorcluster, "FP.State"=w239:T3)
            n78 = Not Equal?(x=w239, y=w237) -> (x != y?=w238:bool)
            n79 = case shown="True" w238 {
              tunnel: [w248 w249] -> w244
              tunnel: w241 -> [w247 w249]
              tunnel: w240 -> [w246 _]
              tunnel: w237 -> [w245 _]
              frame True {
                n80 = invoke class="VI" method="FP.Open"(reference=w246, error in=w247, "State"=w245) -> (error out=w248:errorcluster)  [unwired: 2 in, 4 out]
              }
              frame False {
              }
            }
          }
          frame "Minimize", "Minimized" {
            w250 = T3."Minimized" ("State")
            n81 = property class="VI"(reference=w256, error in=w255) -> (reference out=w253:refnum<vi>, error out=w254:errorcluster, "FP.State"=w252:T3)
            n82 = Not Equal?(x=w252, y=w250) -> (x != y?=w251:bool)
            n83 = case shown="True" w251 {
              tunnel: [w261 w262] -> w257
              tunnel: w254 -> [w260 w262]
              tunnel: w253 -> [w259 _]
              tunnel: w250 -> [w258 _]
              frame True {
                n84 = invoke class="VI" method="FP.Open"(reference=w259, error in=w260, "State"=w258) -> (error out=w261:errorcluster)  [unwired: 2 in, 4 out]
              }
              frame False {
              }
            }
          }
          frame "Maximize", "Maximized" {
            w263 = T3."Maximized" ("State")
            n85 = property class="VI"(reference=w269, error in=w268) -> (reference out=w266:refnum<vi>, error out=w267:errorcluster, "FP.State"=w265:T3)
            n86 = Not Equal?(x=w265, y=w263) -> (x != y?=w264:bool)
            n87 = case shown="True" w264 {
              tunnel: [w274 w275] -> w270
              tunnel: w267 -> [w273 w275]
              tunnel: w266 -> [w272 _]
              tunnel: w263 -> [w271 _]
              frame True {
                n88 = invoke class="VI" method="FP.Open"(reference=w272, error in=w273, "State"=w271) -> (error out=w274:errorcluster)  [unwired: 2 in, 4 out]
              }
              frame False {
              }
            }
          }
        }
        n89 = call <vilib>:"Add State(s) to Queue__JKI_lib_State_Machine.vi"("State(s) in (\"\")"=w210) -> ("States Out"=w209:string)  [unwired: 14 in]
      }
      frame "---------- Macro ----------" {
        # "Do not put any code in this frame.\n(It is a separator no-op. You can make a copy of this frame to create a new Macro frame)"
        n90 = call <vilib>:"Add State(s) to Queue__JKI_lib_State_Machine.vi"("State(s) in (\"\")"=w280) -> ("States Out"=w279:string)  [unwired: 14 in]
      }
      frame "Macro: Initialize" {
        # "Initialization Macro\n(This is called once, when the VI starts)"
        n91 = call <vilib>:"Add State(s) to Queue__JKI_lib_State_Machine.vi"("State(s) in Front (\"\")"="Data: Initialize\nInitialize Core Data\nUI: Initialize\nUI: Front Panel State >> Open\nFastAxis: Open\nSlowAxis: Open\nFastAxis: getTriggerPara", "State(s) in (\"\")"=w286) -> ("States Out"=w285:string)  [unwired: 13 in]
      }
      frame "Macro: Exit" {
        # "Exit Macro\n(This is called once, when the VI exits)"
        n92 = Unbundle By Name(w295) -> ("Core.Close Panel on Exit?"=w294:bool)
        n93 = Select(t="UI: Front Panel State >> Close", s=w294, f="") -> (s? t:f=w291:string)
        n94 = call <vilib>:"Add State(s) to Queue__JKI_lib_State_Machine.vi"("State(s) in Front (\"\")"="FastAxis: Close\nSlowAxis: Close" ("State(s) in Front (\"\")"), "State(s) in (\"\")"=w291, "State(s) at Back (\"\")"="Data: Cleanup\nExit") -> ("States Out"=w289:string)  [unwired: 12 in]
        n95 = call <vilib>:"Add State(s) to Queue__JKI_lib_State_Machine.vi"("State(s) in Front (\"\")"=w289, "State(s) in (\"\")"=w298) -> ("States Out"=w297:string)  [unwired: 13 in]
      }
      frame "---------- FastAxis ----------" {
        # "Template Separator\n(You can make a copy of, or modify, this frame)"
        n96 = call <vilib>:"Add State(s) to Queue__JKI_lib_State_Machine.vi"("State(s) in (\"\")"=w303) -> ("States Out"=w302:string)  [unwired: 14 in]
      }
      frame "FastAxis: Open" {
        # "Open Fast Axis\n(You can make a copy of, or modify, this frame)"
        n97 = property class="KCubeBrushlessControl"(reference="FastAxis", error in=w317, "SerialNumber"="SerialNumber(Fast)") -> (reference out=w319:refnum<k24>, error out=w318:errorcluster)
        n98 = invoke class="KCubeBrushlessControl" method="CreateDevice"(reference=w319, error in=w318) -> (reference out=w316:refnum<k24>, error out=w315:errorcluster)  [unwired: 1 in, 1 out]
        n99 = property class="KCubeBrushlessControl"(reference=w316, error in=w315) -> (reference out=w311:refnum<k24>, error out=w307:errorcluster, "Device"=w308:refnum<k24>)
        n100 = invoke class="KCubeBrushlessMotor" method="GetVelocityParams"(reference=w308, error in=w307, "maxVelocity"=0.0, "acceleration"=0.0) -> (error out=w306:errorcluster, "acceleration"=w305:dbl)  [unwired: 1 in, 3 out]
        n101 = local write "acceleration (mm/s2)"(w305) -> ()
        n102 = Bundle By Name(cluster=w313, "FastAxisSerial"="SerialNumber(Fast)", "NetHandle(Fast)"=w311, "Device(Fast)"=w308) -> (w314:T7)
      }
      frame "FastAxis: ConfigMotion" {
        # "Config fast axis speed\n(You can make a copy of, or modify, this frame)"
        n103 = local read "X speed (mm/s)"() -> (w325:dbl)
        n104 = Unbundle By Name(w328) -> ("Device(Fast)"=w327:refnum<k24>)
        n105 = invoke class="KCubeBrushlessMotor" method="SetVelocityParams"(reference=w327, error in=w323, "maxVelocity"=w325, "acceleration"="acceleration (mm/s2)") -> (error out=w324:errorcluster)  [unwired: 1 in, 4 out]
        n106 = call <vilib>:"Add State(s) to Queue__JKI_lib_State_Machine.vi"("State(s) in (\"\")"=w330) -> ("States Out"=w329:string)  [unwired: 14 in]
      }
      frame "FastAxis: getTriggerPara" {
        # "Get Current Trigger Setting\n(You can make a copy of, or modify, this frame)"
        n107 = Unbundle By Name(w335) -> ("Device(Fast)"=w334:refnum<k24>)
        n108 = stacked-sequence {
          tunnel: w334 -> [w343 w357]
          tunnel: w332 -> [w342 w356]
          tunnel: [_ w344] -> w333
          frame #0 {
            # "get tigger configuration"
            n109 = invoke class="KCubeBrushlessMotor" method="GetTriggerConfigParams"(reference=w343, error in=w342) -> (error out=w340:errorcluster, "GetTriggerConfigParams"=w341:refnum<k24>)  [unwired: 1 in, 1 out]
            n110 = property class="KCubeTriggerConfigParams" props=["Trigger1Mode", "Trigger1Polarity", "Trigger2Mode", "Trigger2Polarity"](reference=w341, error in=w340) -> ("Trigger1Mode"=→"Trigger1Mode":i32, "Trigger1Polarity"=→"Trigger1Polarity":i32)  [unwired: 4 out]
          }
          frame #1 {
            # "get trigger parameter"
            n111 = invoke class="KCubeBrushlessMotor" method="GetTriggerParamsParams"(reference=w357, error in=w356) -> (error out=w354:errorcluster, "GetTriggerParamsParams"=w355:refnum<k24>)  [unwired: 1 in, 1 out]
            n112 = property class="KCubeTriggerParamsParameters"(reference=w355, error in=w354) -> (error out=w344:errorcluster, "CycleCount"=w353:i32, "TriggerCountFwd"=w352:i32, "TriggerCountRev"=w351:i32, "TriggerIntervalFwd"=w350:dbl, "TriggerIntervalRev"=w349:dbl, "TriggerPulseWidth"=w348:i32, "TriggerStartPositionFwd"=w347:dbl, "TriggerStartPositionRev"=w346:dbl)  [unwired: 1 out]
            n113 = Bundle("CycleCount"=w353, "TriggerCountFwd"=w352, "TriggerCountRev"=w351, "TriggerIntervalFwd"=w350, "TriggerIntervalRev"=w349, "TriggerPulseWidth"=w348, "TriggerStartPositionFwd"=w347, "TriggerStartPositionRev"=w346) -> (→"TriggerPara":T1)  [unwired: 1 in]
          }
        }
        n114 = call <vilib>:"Add State(s) to Queue__JKI_lib_State_Machine.vi"("State(s) in (\"\")"=w337) -> ("States Out"=w336:string)  [unwired: 14 in]
      }
      frame "FastAxis: setTriggerMode" {
        w359 = 1 items=["TriggerHigh"=1, "TriggerLow"=2] ("Trigger2Polarity")
        w360 = 0 items=["Disabled"=0, "TrigIN_GPI"=1, "TrigIN_RelativeMove"=2, "TrigIN_AbsoluteMove"=3, "TrigIN_Homed"=4, "TrigIN_Stop"=5, "TrigOUT_GPO"=10, "TrigOUT_InMotion"=11, "TrigOUT_AtMaxVelocity"=12, "TrigOUT_AtPositionFwd"=13, "TrigOUT_AtPositionRev"=14, "TrigOUT_AtPositionBoth"=15, "TrigOut_AtFwdLimit"=16, "TrigOut_AtBwdLimit"=17, "TrigOut_AtLimit"=18] ("Trigger2Mode")
        w366 = 1 items=["TriggerHigh"=1, "TriggerLow"=2] ("Trigger1Polarity")
        w367 = 15 items=["Disabled"=0, "TrigIN_GPI"=1, "TrigIN_RelativeMove"=2, "TrigIN_AbsoluteMove"=3, "TrigIN_Homed"=4, "TrigIN_Stop"=5, "TrigOUT_GPO"=10, "TrigOUT_InMotion"=11, "TrigOUT_AtMaxVelocity"=12, "TrigOUT_AtPositionFwd"=13, "TrigOUT_AtPositionRev"=14, "TrigOUT_AtPositionBoth"=15, "TrigOut_AtFwdLimit"=16, "TrigOut_AtBwdLimit"=17, "TrigOut_AtLimit"=18] ("Trigger1Mode")
        # "Config trigger out \n(You can make a copy of, or modify, this frame)"
        n115 = Unbundle By Name(w371) -> ("Device(Fast)"=w370:refnum<k24>)
        n116 = invoke class="KCubeBrushlessMotor" method="GetTriggerConfigParams"(reference=w370, error in=w361) -> (reference out=w369:refnum<k24>, error out=w364:errorcluster, "GetTriggerConfigParams"=w368:refnum<k24>)  [unwired: 1 in]
        n117 = property class="KCubeTriggerConfigParams"(reference=w368, error in=w364, "Trigger1Mode"=w367, "Trigger1Polarity"=w366, "Trigger2Mode"=w360, "Trigger2Polarity"=w359) -> (reference out=w365:refnum<k24>, error out=w363:errorcluster)
        n118 = invoke class="KCubeBrushlessMotor" method="SetTriggerConfigParams"(reference=w369, error in=w363, "triggerConfigParameters"=w365) -> (error out=w362:errorcluster)  [unwired: 1 in, 3 out]
        n119 = call <vilib>:"Add State(s) to Queue__JKI_lib_State_Machine.vi"("State(s) in (\"\")"=w373) -> ("States Out"=w372:string)  [unwired: 14 in]
      }
      frame "FastAxis: setTriggerPara" {
        # "set trigger parameter\n(You can make a copy of, or modify, this frame)"
        n120 = Unbundle By Name(w395) -> ("Device(Fast)"=w394:refnum<k24>)
        n121 = local read "X step size (um)"() -> (w386:dbl)
        n122 = local read "X scan distance (mm)"() -> (w381:dbl)
        n123 = local read "X0 Position(mm)"() -> (w382:dbl)
        n124 = local read "# of lines"() -> (w391:u32)
        n125 = invoke class="KCubeBrushlessMotor" method="GetTriggerParamsParams"(reference=w394, error in=w375) -> (reference out=w379:refnum<k24>, error out=w392:errorcluster, "GetTriggerParamsParams"=w393:refnum<k24>)  [unwired: 1 in]
        n126 = Divide(x=w386, y=1000.0) -> (x/y=w384:dbl)
        n127 = Divide(x=w391, y=u32 2) -> (x/y=w389:dbl)
        n128 = Add(x=w382, y=w384) -> (x+y=w383:dbl)
        n129 = Divide(x=w381, y=w384) -> (x/y=w387:dbl)
        n130 = Add(x=w382, y=w381) -> (x+y=w380:dbl)
        n131 = property class="KCubeTriggerParamsParameters"(reference=w393, error in=w392, "CycleCount"=w389, "TriggerCountFwd"=w387, "TriggerCountRev"=w387, "TriggerIntervalFwd"=w384, "TriggerIntervalRev"=w384, "TriggerPulseWidth"=50, "TriggerStartPositionFwd"=w383, "TriggerStartPositionRev"=w380) -> (reference out=w377:refnum<k24>, error out=w378:errorcluster)
        n132 = invoke class="KCubeBrushlessMotor" method="SetTriggerParamsParams"(reference=w379, error in=w378, "triggerParamsParameters"=w377) -> (error out=w376:errorcluster)  [unwired: 1 in, 3 out]
        n133 = call <vilib>:"Add State(s) to Queue__JKI_lib_State_Machine.vi"("State(s) in (\"\")"=w397) -> ("States Out"=w396:string)  [unwired: 14 in]
      }
      frame "FastAxis: Close" {
        # "Template Separator\n(You can make a copy of, or modify, this frame)"
        n134 = Unbundle By Name(w402) -> ("NetHandle(Fast)"=w401:refnum<k24>)
        n135 = invoke class="KCubeBrushlessControl" method="CloseDevice"(reference=w401, error in=w400) -> (error out=w399:errorcluster)  [unwired: 1 in, 2 out]
        n136 = call <vilib>:"Simple Error Handler.vi"("error in (no error)"=w399) -> ()  [unwired: 4 in, 5 out]
        n137 = call <vilib>:"Add State(s) to Queue__JKI_lib_State_Machine.vi"("State(s) in (\"\")"=w404) -> ("States Out"=w403:string)  [unwired: 14 in]
      }
      frame "---------- SlowAxis ----------" {
        # "Template Separator\n(You can make a copy of, or modify, this frame)"
        n138 = call <vilib>:"Add State(s) to Queue__JKI_lib_State_Machine.vi"("State(s) in (\"\")"=w409) -> ("States Out"=w408:string)  [unwired: 14 in]
      }
      frame "SlowAxis: Open" {
        # "Template Separator\n(You can make a copy of, or modify, this frame)"
        n139 = property class="KCubeDCServoControl"(reference="SlowAxis", error in=w411, "SerialNumber"="SerialNumber(Slow)") -> (reference out=w421:refnum<k24>, error out=w420:errorcluster)
        n140 = invoke class="KCubeDCServoControl" method="CreateDevice"(reference=w421, error in=w420) -> (reference out=w417:refnum<k24>, error out=w416:errorcluster)  [unwired: 1 in, 1 out]
        n141 = property class="KCubeDCServoControl"(reference=w417, error in=w416) -> (error out=w412:errorcluster, "Device"=w415:refnum<k24>)  [unwired: 1 out]
        n142 = Bundle By Name(cluster=w419, "SlowAxisSerial"="SerialNumber(Slow)", "NetHandle(Slow)"="SlowAxis", "Device(Slow)"=w415) -> (w418:T7)
      }
      frame "SlowAxis: ConfigMotion" {
        # "Template Separator\n(You can make a copy of, or modify, this frame)"
        n143 = call <vilib>:"Add State(s) to Queue__JKI_lib_State_Machine.vi"("State(s) in (\"\")"=w427) -> ("States Out"=w426:string)  [unwired: 14 in]
      }
      frame "SlowAxis: Close" {
        # "Template Separator\n(You can make a copy of, or modify, this frame)"
        n144 = Unbundle By Name(w432) -> ("NetHandle(Slow)"=w431:refnum<k24>)
        n145 = invoke class="KCubeDCServoControl" method="CloseDevice"(reference=w431, error in=w429) -> (error out=w430:errorcluster)  [unwired: 1 in, 2 out]
        n146 = call <vilib>:"Simple Error Handler.vi"("error in (no error)"=w430) -> ()  [unwired: 4 in, 5 out]
        n147 = call <vilib>:"Add State(s) to Queue__JKI_lib_State_Machine.vi"("State(s) in (\"\")"=w434) -> ("States Out"=w433:string)  [unwired: 14 in]
      }
      frame "---------- Scan ----------" {
        # "Template Separator\n(You can make a copy of, or modify, this frame)"
        n148 = call <vilib>:"Add State(s) to Queue__JKI_lib_State_Machine.vi"("State(s) in (\"\")"=w439) -> ("States Out"=w438:string)  [unwired: 14 in]
      }
      frame "Scan: PlanRoute" {
        # "Compute Scan Route\n(You can make a copy of, or modify, this frame)"
        n149 = local read "Y0 Position(mm)"() -> (w446:dbl)
        n150 = local read "# of lines"() -> (w449:u32)
        n151 = Multiply(x=w449, y=u32 2) -> (x*y=w447:u32)
        n152 = for {
          N: w447 -> [_]
          tunnel: [w459] -> w445 mode=indexing
          shift-right: [w455] -> _
          shift-left: w446 -> [w457]
          tunnel: [w455] -> w444 mode=indexing
          i -> [w454]
          n153 = Quotient & Remainder(x=w454, y=2) -> (x-y*floor(x/y)=w458:i32)  [unwired: 1 out]
          n154 = Quotient & Remainder(x=w454, y=4) -> (x-y*floor(x/y)=w452:i32)  [unwired: 1 out]
          n155 = case "X case" shown="0, 3, Default" w452 {
            tunnel: [w468 w474] -> w459
            frame 0, 3, Default {
              n156 = local read "X0 Position(mm)"() -> (w468:dbl)
            }
            frame 1, 2 {
              n157 = local read "X step size (um)"() -> (w473:dbl)
              n158 = local read "X scan distance (mm)"() -> (w476:dbl)
              n159 = local read "X0 Position(mm)"() -> (w477:dbl)
              n160 = Divide(x=w473, y=1000.0) -> (x/y=w471:dbl)
              n161 = Add(x=w477, y=w476) -> (x+y=w475:dbl)
              n162 = Multiply(x=w471, y=10.0) -> (x*y=w469:dbl)
              n163 = Add(x=w475, y=w469) -> (x+y=w474:dbl)
            }
          }
          n164 = case shown="0, Default" w458 {
            tunnel: [w461 0.0 ("x")] -> w456
            tunnel: w454 -> [w464 _]
            frame 0, Default {
              n165 = local read "Y step size (um)"() -> (w466:dbl)
              n166 = Sign(1:w464) -> (0:w463:i32)
              n167 = Divide(x=w466, y=1000.0) -> (x/y=w462:dbl)
              n168 = Multiply(x=w462, y=w463) -> (x*y=w461:dbl)
            }
            frame 1 {
            }
          }
          n169 = Add(x=w456, y=w457) -> (x+y=w455:dbl)
        }
        n170 = Bundle(w445, w444) -> (w441:cluster{dbl[], dbl[]})  [unwired: 1 in]
        "ScanRoute" <- w441
        n171 = Bundle By Name(cluster=w442, "ScanRoute"=w441) -> (w443:T7)
      }
      frame "Scan: StartScan" {
        w484 = T2 {"X"=[], "Y"=[], "Device(Fast)"=refnum, "Device(Slow)"=refnum}  # StartScan
        # "Generate user event to start scan\n(You can make a copy of, or modify, this frame)"
        n172 = Unbundle By Name(w482) -> ("ScanRoute"=w490:cluster{dbl[], dbl[]}, "Device(Fast)"=w487:refnum<k24>, "Device(Slow)"=w486:refnum<k24>)
        n173 = Unbundle(w490) -> (w489:dbl[], w488:dbl[])
        n174 = Bundle By Name(cluster=w484, "X"=w489, "Y"=w488, "Device(Fast)"=w487, "Device(Slow)"=w486) -> (w485:T2)
        n175 = Generate User Event(priority (normal)=usereventprio."high priority", user event=w481, event data cluster=w485, error in=w479) -> (error out=w480:errorcluster)  [unwired: 1 out]
        n176 = call <vilib>:"Add State(s) to Queue__JKI_lib_State_Machine.vi"("State(s) in (\"\")"=w492) -> ("States Out"=w491:string)  [unwired: 14 in]
      }
      frame "Scan: SaveInfo" {
        # "save scan information to encoder TDMS\n(You can make a copy of, or modify, this frame)"
        n177 = call "EncoderTDMS_Path.vi"("error in (no error)"=w493, "Operation (Read)"=enum16{"Write", "Read"}."Read") -> ("error out"=w511:errorcluster, "Path Out"=w512:path)  [unwired: 8 in]
        n178 = TDMS Open(8:w511, 10:T6."open" ("operation (0:open)"), 11:w512) -> (0:w508:errorcluster, 3:w509:refnum<k34>)  [unwired: 4 in]
        n179 = local read "# of lines"() -> (w498:u32)
        n180 = local read "X step size (um)"() -> (w501:dbl)
        n181 = local read "Y step size (um)"() -> (w500:dbl)
        n182 = local read "X0 Position(mm)"() -> (w505:dbl)
        n183 = local read "Y0 Position(mm)"() -> (w504:dbl)
        n184 = local read "X speed (mm/s)"() -> (w499:dbl)
        n185 = local read "X scan distance (mm)"() -> (w503:dbl)
        n186 = local read "Y scan distance (mm)"() -> (w502:dbl)
        n187 = Build Array(w505, w504, w503, w502, w501, w500, w499, w498) -> (w497:dbl[])
        n188 = TDMS Set Properties(5:w497, 7:string[] ["X0 (mm)", "Y0 (mm)", "X scan distance (mm)", "Y scan distance (mm)", "X step size (um)", "Y step size (um)", "X speed (mm/s)", "num of lines"] ("property names"), 8:w508, 10:"Encoder" ("group name"), 11:w509) -> (0:w495:errorcluster, 3:w496:refnum<k34>)  [unwired: 1 in, 2 out]
        n189 = TDMS Close(8:w495, 11:w496) -> (0:w494:errorcluster)  [unwired: 1 out]
        n190 = call <vilib>:"Add State(s) to Queue__JKI_lib_State_Machine.vi"("State(s) in (\"\")"=w517) -> ("States Out"=w516:string)  [unwired: 14 in]
      }
      frame "---------- FLIm ----------" {
        # "Template Separator\n(You can make a copy of, or modify, this frame)"
        n191 = call <vilib>:"Add State(s) to Queue__JKI_lib_State_Machine.vi"("State(s) in (\"\")"=w522) -> ("States Out"=w521:string)  [unwired: 14 in]
      }
      frame "FLIm: remoteStart" {
        # "remote start FLIm\n(You can make a copy of, or modify, this frame)"
        n192 = call "RemoteEventFGV.vi"("Error In"=w524, "Operation (Read)"=enum16{"Read", "Write"}."Read") -> ("Error Out"=w526:errorcluster, "Remote Event out"=w530:T9)  [unwired: 8 in]
        n193 = Unbundle By Name(w530) -> ("remote start event"=w529:refnum<user-event>)
        n194 = Generate User Event(priority (normal)=usereventprio."high priority", user event=w529, event data cluster=FALSE ("event data"), error in=w526) -> (error out=w525:errorcluster)  [unwired: 1 out]
      }
      frame "FLIm: remoteStop" {
        # "remote stop FLIm\n(You can make a copy of, or modify, this frame)"
        n195 = call "RemoteEventFGV.vi"("Error In"=w535, "Operation (Read)"=enum16{"Read", "Write"}."Read") -> ("Error Out"=w537:errorcluster, "Remote Event out"=w540:T9)  [unwired: 8 in]
        n196 = Unbundle By Name(w540) -> ("remote stop event"=w539:refnum<user-event>)
        n197 = Generate User Event(user event=w539, event data cluster=FALSE ("event data"), error in=w537) -> (error out=w536:errorcluster)  [unwired: 1 in, 1 out]
        n198 = call <vilib>:"Add State(s) to Queue__JKI_lib_State_Machine.vi"("State(s) in (\"\")"=w544) -> ("States Out"=w543:string)  [unwired: 14 in]
      }
      frame "---------- Utility ----------" {
        # "Template Separator\n(You can make a copy of, or modify, this frame)"
        n199 = call <vilib>:"Add State(s) to Queue__JKI_lib_State_Machine.vi"("State(s) in (\"\")"=w549) -> ("States Out"=w548:string)  [unwired: 14 in]
      }
      frame "Utility: Dewell" {
        # "Template Separator\n(You can make a copy of, or modify, this frame)"
        n200 = Decimal String To Number(string=w552) -> (number=w551:i32)  [unwired: 2 in, 1 out]
        n201 = Wait (ms)(milliseconds to wait=w551) -> ()  [unwired: 1 out]
        n202 = call <vilib>:"Add State(s) to Queue__JKI_lib_State_Machine.vi"("State(s) in (\"\")"=w556) -> ("States Out"=w555:string)  [unwired: 14 in]
      }
      frame "---------- New Category ----------" {
        # "Template Separator\n(You can make a copy of, or modify, this frame)"
        n203 = call <vilib>:"Add State(s) to Queue__JKI_lib_State_Machine.vi"("State(s) in (\"\")"=w561) -> ("States Out"=w560:string)  [unwired: 14 in]
      }
      frame "New Category: 1" {
        # "Your code here.\n(You can make a copy of, or modify, this frame)"
        n204 = call <vilib>:"Add State(s) to Queue__JKI_lib_State_Machine.vi"("State(s) in (\"\")"=w566) -> ("States Out"=w565:string)  [unwired: 14 in]
      }
      frame "New Category: 2" {
        # "Your code here.\n(You can make a copy of, or modify, this frame)"
        n205 = call <vilib>:"Add State(s) to Queue__JKI_lib_State_Machine.vi"("State(s) in (\"\")"=w571) -> ("States Out"=w570:string)  [unwired: 14 in]
      }
    }
  }
  n206 = while {
    tunnel: w17 -> [w575]
    tunnel: [w573] -> w12
    tunnel: w4 -> [w572]
    stop <- w574 stop-if-true
    n207 = event shown="[2] <StartScan>: User Event" {
      selector: w575 -> [_ _ _]
      dyn-events: [_ _ _] -> w573
      timeout: 30 -> [_ _ _]
      tunnel: [FALSE ("Quit") TRUE ("Quit") _] -> w574
      tunnel: w572 -> [_ _ w579]
      event Timeout {
        n208 = event-data() -> ()  [unwired: 1 in, 3 out]
      }
      event User Event {
        n209 = event-data() -> ()  [unwired: 1 in, 5 out]
      }
      event User Event {
        w581 = 0.0  # Y
        w582 = 0.0  # X
        n210 = event-data() -> ("X"=w586:dbl[], "Y"=w585:dbl[], "Device(Fast)"=w587:refnum<k24>, "Device(Slow)"=w583:refnum<k24>)  [unwired: 1 in, 4 out]
        n211 = for {
          tunnel: w587 -> [w601]
          tunnel: w586 -> [w592] mode=indexing
          tunnel: w585 -> [w591] mode=indexing
          shift-right: [w597] -> w580
          shift-left: errorcluster {"status"=FALSE, "code"=0, "source"=""} ("error constant") -> [w600]
          tunnel: w583 -> [w599]
          shift-right: [w592] -> _
          shift-left: w582 -> [w595]
          shift-right: [w591] -> _
          shift-left: w581 -> [w594]
          n212 = Not Equal?(x=w595, y=w592) -> (x != y?=w596:bool)
          n213 = Not Equal?(x=w591, y=w594) -> (x != y?=w593:bool)
          n214 = case shown="True" w596 {
            tunnel: w601 -> [_ w617]
            tunnel: w600 -> [w610 w616]
            tunnel: [w610 w613] -> w598
            tunnel: w592 -> [_ w612]
            frame False {
              # "if same x, do nothing"
            }
            frame True {
              # "if different x, move"
              n215 = invoke class="KCubeBrushlessMotor" method="SetMoveAbsolutePosition"(reference=w617, error in=w616, "position"=w612) -> (reference out=w615:refnum<k24>, error out=w614:errorcluster)  [unwired: 1 in, 2 out]
              n216 = invoke class="KCubeBrushlessMotor" method="MoveAbsolute"(reference=w615, error in=w614, "waitTimeout"=10000) -> (error out=w613:errorcluster)  [unwired: 1 in, 3 out]
            }
          }
          n217 = case shown="True" w593 {
            tunnel: w599 -> [_ w609]
            tunnel: w598 -> [w602 w608]
            tunnel: [w602 w605] -> w597
            tunnel: w591 -> [_ w604]
            frame False {
              # "If same y, do nothing"
            }
            frame True {
              # "if different y, move"
              n218 = invoke class="KCubeDCServo" method="SetMoveAbsolutePosition"(reference=w609, error in=w608, "position"=w604) -> (reference out=w607:refnum<k24>, error out=w606:errorcluster)  [unwired: 1 in, 2 out]
              n219 = invoke class="KCubeDCServo" method="MoveAbsolute"(reference=w607, error in=w606, "waitTimeout"=10000) -> (error out=w605:errorcluster)  [unwired: 1 in, 3 out]
            }
          }
        }
        n220 = call <vilib>:"Simple Error Handler.vi"("error in (no error)"=w580) -> ()  [unwired: 4 in, 5 out]
        n221 = flat-sequence {
          tunnel: w580 -> [_]
          tunnel: w579 -> [w590]
          frame #0 {
            n222 = Generate User Event(priority (normal)=usereventprio."high priority", user event=w590, event data cluster=FALSE ("event data")) -> ()  [unwired: 1 in, 2 out]
          }
        }
      }
    }
  }
  n223 = Destroy User Event(user event=w4, error in=w6) -> (error out=w7:errorcluster)
  n224 = Destroy User Event(user event=w11, error in=w7) -> (error out=w9:errorcluster)
  n225 = Destroy User Event(user event=w10, error in=w9) -> (error out=w8:errorcluster)
  n226 = Unregister For Events(event registration refnum=w12, error in=w8) -> (error out=w2:errorcluster)
  n227 = Unregister For Events(event registration refnum=w1, error in=w2) -> (error out=→"error out":errorcluster)
